vi "PAN_VAR_Status.vi"(8 "error in (no error)":errorcluster, 9 "action":enum16{"read", "write", "set_ref"}(ring)=enum."write", 10 "status in":string, 11 "status":refnum<vi>) -> (0 "error out":errorcluster, 2 "status out":string)   [LabVIEW 2016]
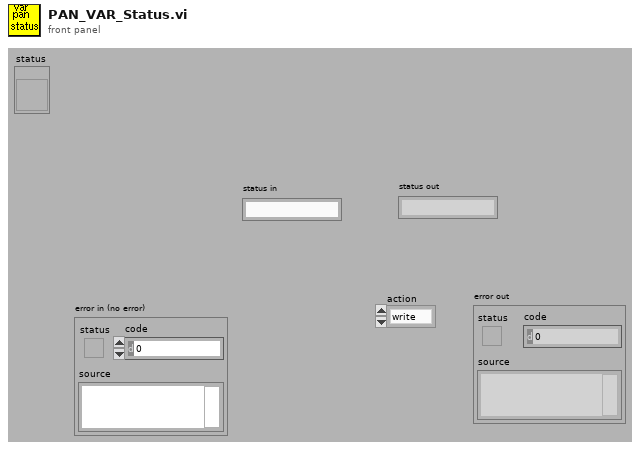
[diagram p1: front panel]
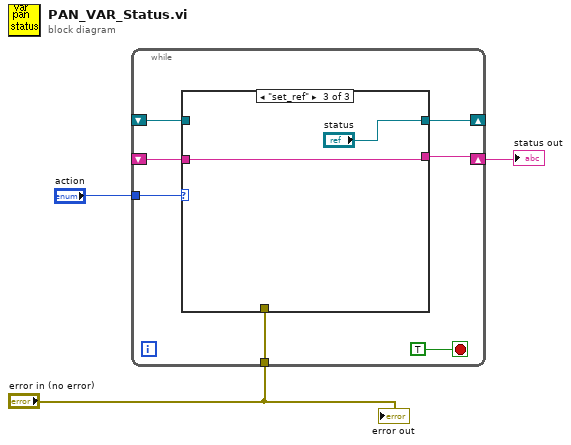
[diagram p0: block diagram]
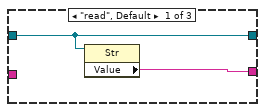
[diagram p2: hidden frame]
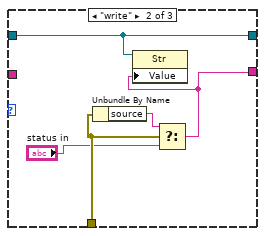
[diagram p3: hidden frame]
diagram:
  n1 = while {
    tunnel: "action" -> [w9]
    shift-right: [w8] -> w2
    shift-left: _ -> [w7]
    tunnel: "error in (no error)" -> [w6]
    shift-right: [w5] -> _
    shift-left: _ -> [w4]
    stop <- TRUE stop-if-true
    n2 = case shown="\"set_ref\"" w9 {
      tunnel: [w11 w13 w18] -> w8
      tunnel: w7 -> [_ _ w18]
      tunnel: w6 -> [_ w17 _]
      tunnel: [w12 w14 "status"] -> w5
      tunnel: w4 -> [w12 w14 _]
      frame "read", Default {
        n3 = property class="Str"(reference=w12) -> ("Value"=w11:string)  [unwired: 1 in, 2 out]
      }
      frame "write" {
        n4 = Unbundle By Name(w17) -> ("source"=w16:string)
        n5 = Select(t=w16, s=w17, f="status in") -> (s? t:f=w13:string)
        n6 = property class="Str"(reference=w14, "Value"=w13) -> ()  [unwired: 1 in, 2 out]
      }
      frame "set_ref" {
      }
    }
  }
  "status out" <- w2
  "error out" <- "error in (no error)"
